vi "inst.SpareRelays (DPDT).vi"(7 "unit ID":u8, 8 "error in (no error)":errorcluster, 10 "SpareRelays":bool[](array[boolean])=[FALSE, FALSE, FALSE, FALSE, FALSE, FALSE, FALSE, FALSE, FALSE, FALSE, FALSE, FALSE, FALSE, FALSE, FALSE], 11 "Modbus Master in":refnum<class "Modbus Master.lvclass">) -> (0 "error out":errorcluster, 3 "Modbus Master out":refnum<class "Modbus Master.lvclass">)   [LabVIEW 2018, in "MB Relay.lvlib"]
uses:
  MB Relay.lvlib
  <vilib>/NI/Modbus Library/API/Master/Modbus Master.lvclass
  type defs/FGV enum.ctl
  type defs/FGV data cluster.ctl
  type defs/MB relays _InstrumentType.ctl
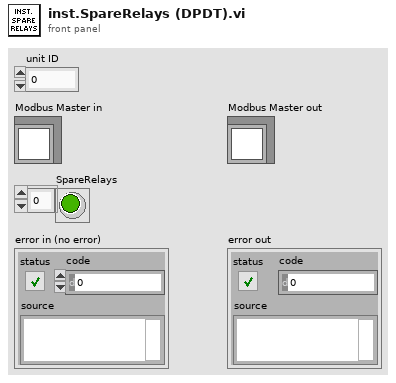
[diagram p1: front panel]
types:
  T1 = typedef "MB Relay.lvlib/MB relays _InstrumentType.ctl" = enum16{"counter", "demux1_10(x6)", "mux10_1(x6)", "mux6_1(3wires)", "MB_Relay_01(eMICs)", "SpareRelays(DPDT)", "Optos", "Inputs", "DMM I 0.5", "SpareRelays (SPDT)", "SC enable"}
  T2 = typedef "MB Relay.lvlib/FGV data cluster.ctl" = cluster{"demux1_10(x6)_encode":enum16{"demux1_10_channel0", "demux1_10_channel1", "demux1_10_channel2", "demux1_10_channel3", "demux1_10_channel4", "demux1_10_channel5", "demux1_10_channel6", "demux1_10_channel7", "demux1_10_channel8", "demux1_10_channel9", "demux1_10_channel10"}, "mux10_1(x6)_encode":enum16{"mux10_1_channel0", "mux10_1_channel1", "mux10_1_channel2", "mux10_1_channel3", "mux10_1_channel4", "mux10_1_channel5", "mux10_1_channel6", "mux10_1_channel7", "mux10_1_channel8", "mux10_1_channel9", "mux10_1_channel10"}, "MB Relay01":bool[], "SpareRelays (DPDT)":bool[], "mux6_1(3wires)_encode":enum16{"mux6-1_channel0", "mux6_1_channel1_0", "mux6_1_channel1_1", "mux6-1_channel1_2", "mux6_1_channel1_3", "mux6_1_channel2_0", "mux6_1_channel2_1", "mux6_1_channel2_2", "mux6_1_channel2_3", "mux6_1_channel3_0", "mux6_1_channel3_1", "mux6_1_channel3_2", "mux6_1_channel3_3", "mux6_1_channel4_0", "mux6_1_channel4_1", "mux6_1_channel4_2", "mux6_1_channel4_3", "mux6_1_channel5_0", "mux6_1_channel5_1", "mux6_1_channel5_2", "mux6_1_channel5_3", "mux6_1_channel6_0", "mux6_1_channel6_1", "mux6_1_channel6_2", "mux6_1_channel6_3"}, "mux2-1(DMM I) encode":enum16{"DMM I (0.5)", "DMM I (12)"}, "5V enable":bool, "SpareRelays (SPDT)":bool[]}
  T3 = typedef "MB Relay.lvlib/FGV enum.ctl" = enum16{"Write", "Read", "All OFF", "All ON"}
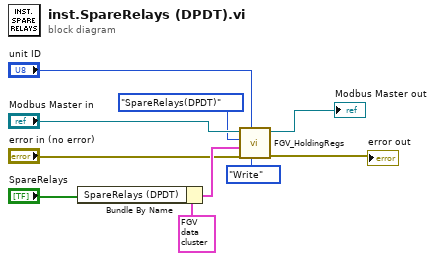
[diagram p0: block diagram]
diagram:
  n1 = Bundle By Name(cluster=T2 {"demux1_10(x6)_encode"=enum."demux1_10_channel0", "mux10_1(x6)_encode"=enum."mux10_1_channel0", "MB Relay01"=[], "SpareRelays (DPDT)"=[], "mux6_1(3wires)_encode"=enum."mux6-1_channel0", "mux2-1(DMM I) encode"=enum."DMM I (0.5)", "5V enable"=FALSE, "SpareRelays (SPDT)"=[FALSE, FALSE, FALSE, FALSE, FALSE, FALSE, FALSE, FALSE, FALSE, FALSE, FALSE, FALSE, FALSE, FALSE, FALSE, FALSE, FALSE, FALSE, FALSE, FALSE, FALSE, FALSE, FALSE, FALSE, FALSE, FALSE, FALSE, FALSE, FALSE, FALSE, FALSE, FALSE]} ("FGV_ data cluster"), "SpareRelays (DPDT)"="SpareRelays") -> (w8:T2)
  n2 = call "FGV_HoldingRegs.vi"("FGV_enum"=FGV_enum."Write", "unit ID"="unit ID", "error in (no error)"="error in (no error)", "FGV_ data cluster"=w8, "Instruments"=MB_relays__InstrumentType."SpareRelays(DPDT)", "Modbus master in"="Modbus Master in") -> ("error out"=→"error out":errorcluster, "Modbus master out"=→"Modbus Master out":refnum<class "Modbus Master.lvclass">)  [unwired: 3 in, 1 out]
